vi "Intake_Test_code.vi"(1 "Ramp Rate \n%/Sec":dbl, 2 "Low Speed":dbl, 3 "Disable T/F":bool, 4 "High Speed":dbl) -> ()   [LabVIEW 2019]
uses:
  ArgosLib/ArgosLib.lvlib
  <vilib>/Rock Robotics/WPI/Joystick/WPI_JoystickDeviceEnum.ctl
  <vilib>/Rock Robotics/WPI/Joystick/WPI_JoystickDevRef.ctl
panel:
  in  "Joystick_In":T1
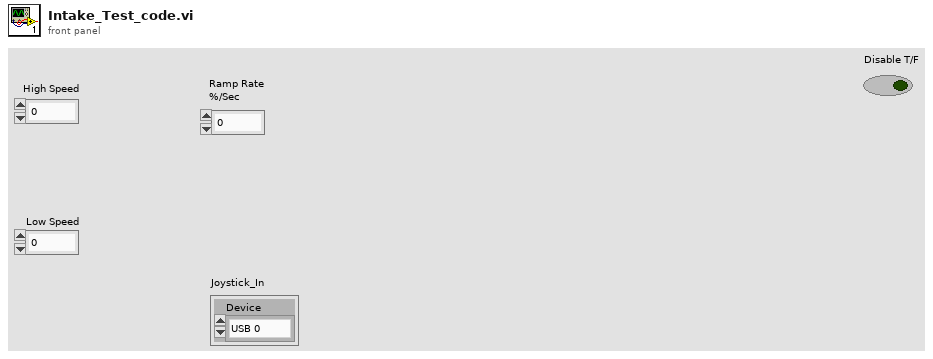
[diagram p1: front panel]
types:
  T1 = typedef "WPI_JoystickDevRef.ctl" = cluster{"Device":T2}
  T2 = typedef "WPI_JoystickDeviceEnum.ctl" = enum16{"USB 0", "USB 1", "USB 2", "USB 3", "USB 4", "USB 5"}
  T3 = typedef "XBoxButtons_Type.ctl" = cluster{"A":bool, "B":bool, "X":bool, " Y":bool, "LB":bool, " RB":bool, "Left_Thumb_Button":bool, "Right_Thumb_Button":bool, "Back":bool, "Start":bool, "Top":bool, "Right":bool, "Bottom":bool, "Left":bool}
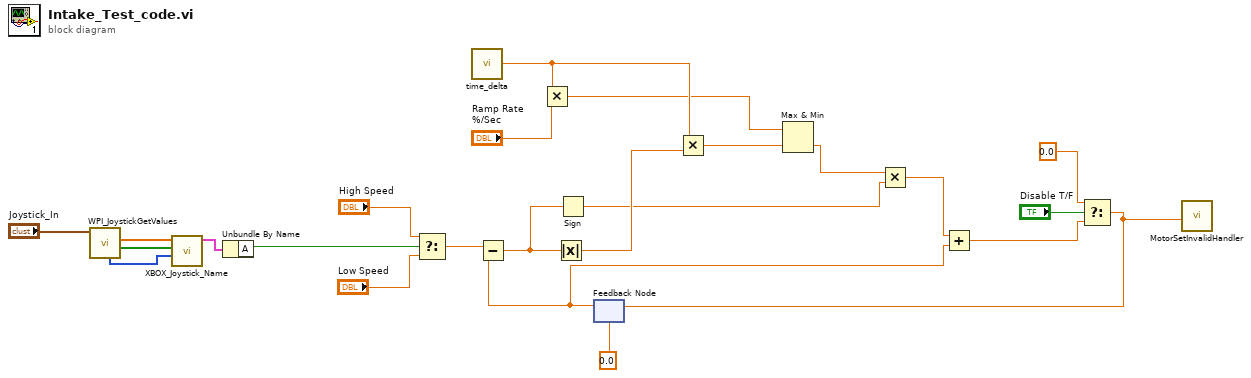
[diagram p0: block diagram]
diagram:
  n1 = call <vilib>:"WPI_JoystickGetValues.vi"("JoystickDevRef"="Joystick_In") -> ("Buttons"=w5:bool[], "Axes"=w6:dbl[], "POVs"=w4:i16[])  [unwired: 6 in, 2 out]
  n2 = call "XBOX_Joystick_Name.vi"("POVs"=w4, "Buttons"=w5, "Axes"=w6) -> ("Named Buttons"=w2:T3)  [unwired: 7 in, 1 out]
  n3 = Unbundle By Name(w2) -> ("A"=w1:bool)
  n4 = Select(t="High Speed", s=w1, f="Low Speed") -> (s? t:f=w22:dbl)
  n5 = call "time_delta.vi"() -> ("dt (s)"=w18:dbl)  [unwired: 1 in]
  n6 = Multiply(x=w18, y="Ramp Rate \n%/Sec") -> (x*y=w17:dbl)
  n7 = feedback #1(0.0) -> (w8:dbl)
  n8 = Subtract(x=w22, y=w8) -> (x-y=w21:dbl)
  n9 = Absolute Value(x=w21) -> (abs(x)=w20:dbl)
  n10 = Sign(1:w21) -> (0:w14:dbl)
  n11 = Multiply(x=w18, y=w20) -> (x*y=w16:dbl)
  n12 = Max & Min(x=w17, y=w16) -> (min(x,y)=w15:dbl)  [unwired: 1 out]
  n13 = Multiply(x=w15, y=w14) -> (x*y=w9:dbl)
  n14 = Add(x=w9, y=w8) -> (x+y=w10:dbl)
  n15 = Select(t=0.0, s="Disable T/F", f=w10) -> (s? t:f=w7:dbl)
  n16 = feedback-in #1(w7) -> ()
  n17 = call "MotorSetInvalidHandler.vi"("Output"=w7) -> ()  [unwired: 8 in, 3 out]
